vi "exec.vi"(8 "error in (no error)":errorcluster, 10 "context":refnum<class "Context.lvclass">, 11 "StopAutomatedTest in":refnum<class "StopAutomatedTest.lvclass">) -> (0 "error out":errorcluster, 2 "context 2":refnum<class "Context.lvclass">, 3 "StopAutomatedTest out":refnum<class "StopAutomatedTest.lvclass">)   [LabVIEW 2013, in "StopAutomatedTest.lvclass"]
uses:
  StopAutomatedTest.lvclass
  Context/Context.lvclass
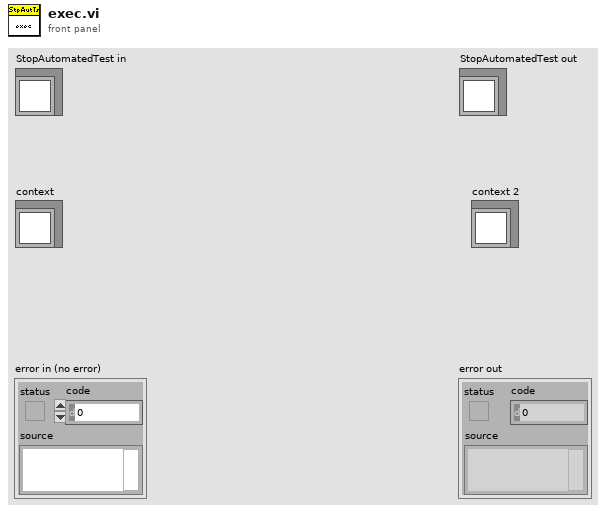
[diagram p1: front panel]
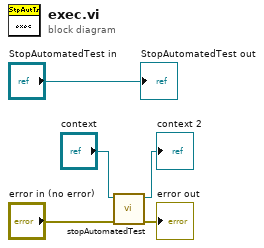
[diagram p0: block diagram]
diagram:
  n1 = call "stopAutomatedTest.vi"("error in (no error)"="error in (no error)", "Context in"="context") -> ("error out"=→"error out":errorcluster, "Context out"=→"context 2":refnum<class "Context.lvclass">)  [unwired: 8 in]
  "StopAutomatedTest out" <- "StopAutomatedTest in"
